vi "RunOperation.vi"(10 "Inputs":string[](array[string]), 11 "VIPMUninstallPackage in":refnum<class "VIPMUninstallPackage.lvclass">) -> (1 "Output/Failure":string, 2 "CLI Process Return Code":i32, 3 "VIPMUninstallPackage out":refnum<class "VIPMUninstallPackage.lvclass">)   [LabVIEW 2014, in "VIPMUninstallPackage.lvclass"]
uses:
  <nishared>/LabVIEW CLI/Operations/VIPMUninstallPackage/VIPMUninstallPackage.lvclass
  <nishared>/LabVIEW CLI/Operations/VIPMUninstallPackage/VIPMUninstallPackage.lvclass/VIPMUninstallPackage.ctl
  <vilib>/JKI/VIPM API/VIPM API_vipm_api.lvlib
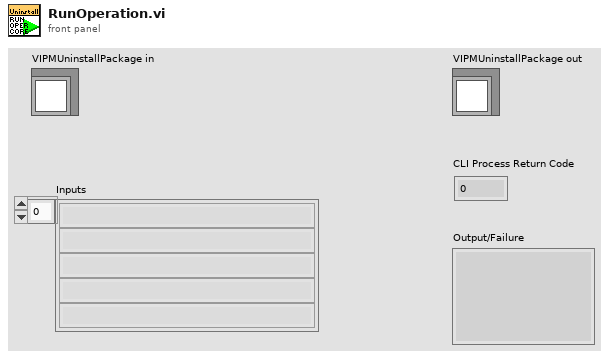
[diagram p1: front panel]
types:
  T1 = typedef "VIPM API_vipm_api.lvlib/Library Contents Cluster_vipm_api.ctl" = cluster{"Package Name":string, "Version":string, "Display Name":string, "Repository Name":string, "Company Name":string, "License Type":string, "Installed":bool, "Deprecated":bool, "Dependency or Conflict Problem":bool, "Downloaded":bool}
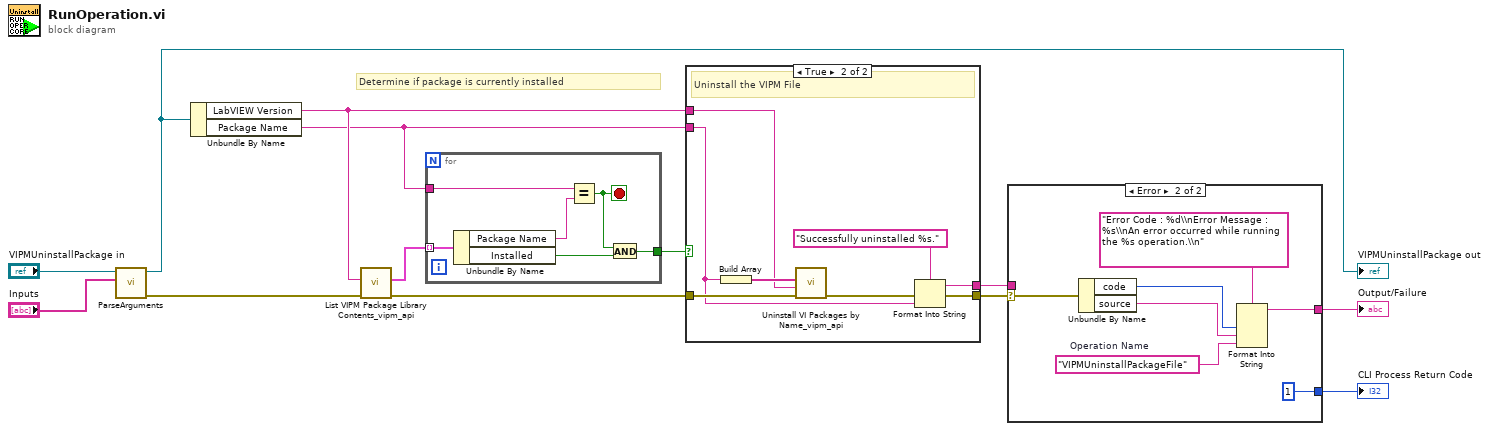
[diagram p0: block diagram]
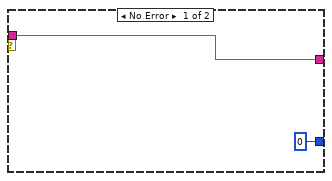
[diagram p2: hidden frame]
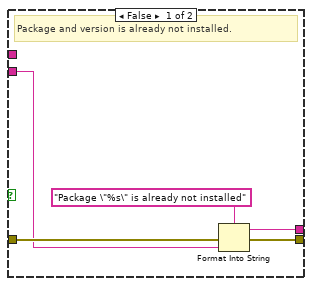
[diagram p3: hidden frame]
diagram:
  # "Determine if package is currently installed"
  n1 = call <nishared>:"ParseArguments.vi"("Inputs"="Inputs", "VIPMUninstallPackage in"="VIPMUninstallPackage in") -> ("error out"=w10:errorcluster, "VIPMUninstallPackage out"=w11:refnum<class "VIPMUninstallPackage.lvclass">)  [unwired: 8 in]
  "VIPMUninstallPackage out" <- w11
  n2 = Unbundle By Name(w11) -> ("LabVIEW Version"=w8:string, "Package Name"=w6:string)
  n3 = call <vilib>:"List VIPM Package Library Contents_vipm_api.vi"("error in (no error)"=w10, "LabVIEW Version"=w8) -> ("error out"=w9:errorcluster, "Library Contents []"=w7:T1[])  [unwired: 8 in]
  n4 = for {
    tunnel: w7 -> [w19] mode=indexing
    tunnel: w6 -> [w18]
    tunnel: [w14] -> w5
    stop <- w16 stop-if-true
    n5 = Unbundle By Name(w19) -> ("Package Name"=w17:string, "Installed"=w15:bool)
    n6 = Equal?(x=w18, y=w17) -> (x = y?=w16:bool)
    n7 = And(x=w16, y=w15) -> (x .and. y?=w14:bool)
  }
  n8 = case shown="True" w5 {
    tunnel: w9 -> [w24 w31]
    tunnel: w8 -> [_ w30]
    tunnel: w6 -> [w20 w25]
    tunnel: [w22 w27] -> w2
    tunnel: [w21 w26] -> w1
    frame False {
      # "Package and version is already not installed."
      n9 = Format Into String(format string="Package \"%s\" is already not installed", error in=w24, w20) -> (resulting string=w21:string, error out=w22:errorcluster)  [unwired: 1 in]
    }
    frame True {
      # "Uninstall the VIPM File"
      n10 = Build Array(w25) -> (w32:string[])
      n11 = call <vilib>:"Uninstall VI Packages by Name_vipm_api.vi"("error in (no error)"=w31, "LabVIEW Version"=w30, "Package Names to Uninstall []"=w32) -> ("error out"=w28:errorcluster)  [unwired: 8 in]
      n12 = Format Into String(format string="Successfully uninstalled %s.", error in=w28, w25) -> (resulting string=w26:string, error out=w27:errorcluster)  [unwired: 1 in]
    }
  }
  n13 = case shown="Error" w2 {
    selector: w2 -> [_ w41]
    tunnel: [w33 w36] -> w3
    tunnel: [0 ("CLI Process Return Code") 1 ("CLI Process Return Code")] -> w4
    tunnel: w1 -> [w33 _]
    frame No Error {
    }
    frame Error {
      w37 = "VIPMUninstallPackageFile"  # Operation Name
      n14 = Unbundle By Name(w41) -> ("code"=w40:i32, "source"=w39:string)
      n15 = Format Into String(format string="Error Code : %d\\nError Message : %s\\nAn error occurred while running the %s operation.\\n" ("Format Error Output String"), w40, w39, w37) -> (resulting string=w36:string)  [unwired: 2 in, 1 out]
    }
  }
  "CLI Process Return Code" <- w4
  "Output/Failure" <- w3
